vi "Actor Core.vi"(8 "error in (no error)":errorcluster, 11 "Websocket Server in":refnum<class "Websocket Server.lvclass">) -> (0 "error out":errorcluster, 3 "Websocket Server out":refnum<class "Websocket Server.lvclass">)   [LabVIEW 2016, in "Stream Mediator.lvlib" / "Websocket Server.lvclass"]
doc: "--\nCopyright © 2017 Composed SystemsI All rights reserved.\n\nAuthor: Jon McBee <jon.mcbee@composed.io>\n\nThis library is provided \"AS IS\" ,WITHOUT WARRANTIES OR\nCONDITIONS OF ANY KIND, either express or implied.\n\nComposed Systems -- composed.io\n\nStream 0.0.1.1\nJon McBee - Composed Systems\nCopyright (c) 2017, Composed Systems"
uses:
  <userlib>/Composed Systems/Stream/Mediator/Classes/Websocket Server Actor/Websocket Server/Websocket Server.lvclass
  C:/Program Files (x86)/National Instruments/LabVIEW 2016/user.lib/Composed Systems/Stream/Mediator/Classes/Mediated Asynchronous Actor/Mediated Asynchronous Actor.lvclass
  <userlib>/Composed Systems/Stream/Mediator/Classes/Message Transport Queue/Message Transport Queue.lvclass
  <userlib>/Composed Systems/Stream/Mediator/Classes/Websocket Server Actor/Websocket Server/Websocket Server.lvclass/Websocket Server.ctl
  <userlib>/Composed Systems/Stream/Mediator/Classes/Mediated Asynchronous Actor/Mediated Asynchronous Actor.lvclass
  <userlib>/Composed Systems/Stream/Mediator/Classes/Websocket Server Actor/Websocket Server Msgs/Launch Client Handler Actor Msg/Launch Client Handler Actor Msg.lvclass
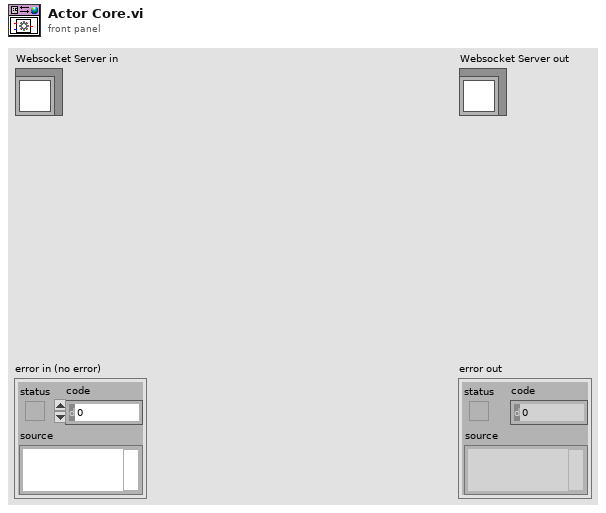
[diagram p1: front panel]
types:
  T1 = cluster{"Self Enqueuer":refnum<class "Message Transport Queue.lvclass">, "Listen Port":u16, "Listener ID":refnum<k5>}
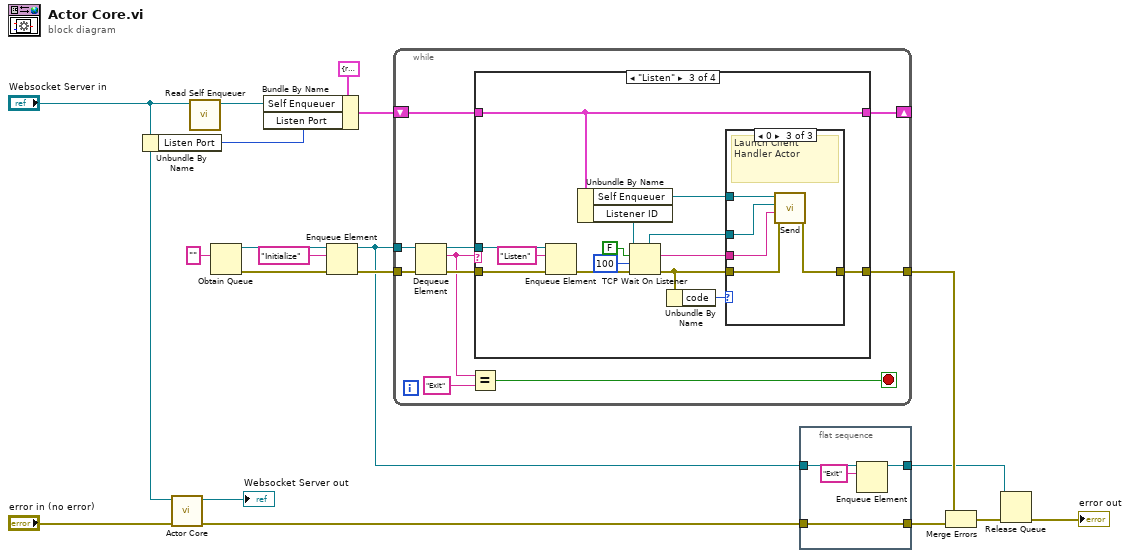
[diagram p0: block diagram]
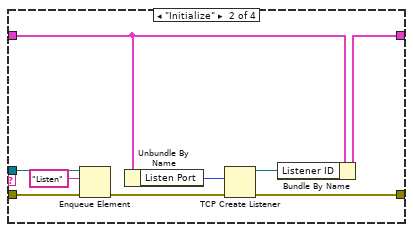
[diagram p3: hidden frame]
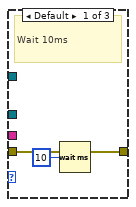
[diagram p4: hidden frame]
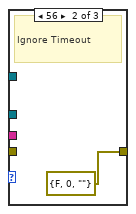
[diagram p5: hidden frame]
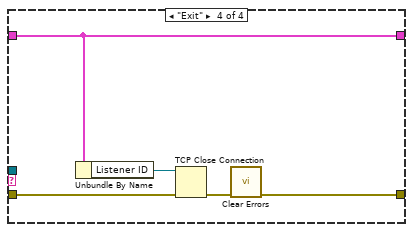
[diagram p6: hidden frame]
diagram:
  n1 = Unbundle By Name("Websocket Server in") -> ("Listen Port"=w9:u16)
  n2 = call-parent "Actor Core.vi"("error in (no error)"="error in (no error)", "Mediated Asynchronous Actor in"="Websocket Server in") -> ("error out"=w13:errorcluster, "Mediated Asynchronous Actor out"=→"Websocket Server out":refnum<class "Websocket Server.lvclass">)  [unwired: 8 in]
  n3 = call <userlib>:"Read Self Enqueuer.vi"("Mediated Asynchronous Actor in"="Websocket Server in") -> ("Self Enqueuer"=w2:refnum<class "Message Transport Queue.lvclass">)  [unwired: 10 in]
  n4 = Obtain Queue(element data type="") -> (queue out=w14:refnum<queue>, error out=w17:errorcluster)  [unwired: 4 in, 1 out]
  n5 = Bundle By Name(cluster=T1 {"Self Enqueuer"=refnum, "Listen Port"=0, "Listener ID"=refnum}, "Self Enqueuer"=w2, "Listen Port"=w9) -> (w8:T1)
  n6 = Enqueue Element(queue=w14, element="Initialize", error in (no error)=w17) -> (queue out=w11:refnum<queue>, error out=w16:errorcluster)  [unwired: 1 in, 1 out]
  n7 = while {
    tunnel: w11 -> [w29]
    tunnel: w16 -> [w28]
    shift-right: [w24] -> _
    shift-left: w8 -> [w25]
    tunnel: [w20] -> w7
    stop <- w21 stop-if-true
    n8 = Dequeue Element(queue=w29, error in (no error)=w28) -> (queue out=w27:refnum<queue>, element=w23:string, error out=w26:errorcluster)  [unwired: 1 in, 1 out]
    n9 = Equal?(x=w23, y="Exit") -> (x = y?=w21:bool)
    n10 = case shown="\"Listen\"" w23 {
      tunnel: w27 -> [_ w40 w51 _]
      tunnel: w26 -> [w30 w39 w52 w66]
      tunnel: w25 -> [w31 w33 w48 w64]
      tunnel: [w31 w32 w48 w64] -> w24
      tunnel: [w30 w36 w44 w65] -> w20
      frame "", Default {
      }
      frame "Initialize" {
        n11 = Enqueue Element(queue=w40, element="Listen", error in (no error)=w39) -> (error out=w37:errorcluster)  [unwired: 1 in, 2 out]
        n12 = Unbundle By Name(w33) -> ("Listen Port"=w35:u16)
        n13 = TCP Create Listener(8:w37, 10:w35) -> (0:w36:errorcluster, 3:w34:refnum<k5>)  [unwired: 3 in, 1 out]
        n14 = Bundle By Name(cluster=w33, "Listener ID"=w34) -> (w32:T1)
      }
      frame "Listen" {
        n15 = Enqueue Element(queue=w51, element="Listen", error in (no error)=w52) -> (error out=w49:errorcluster)  [unwired: 1 in, 2 out]
        n16 = Unbundle By Name(w48) -> ("Self Enqueuer"=w43:refnum<class "Message Transport Queue.lvclass">, "Listener ID"=w47:refnum<k5>)
        n17 = TCP Wait On Listener(8:w49, 9:100 ("timeout ms (wait forever: -1)"), 10:FALSE ("resolve remote address (T)"), 11:w47) -> (0:w45:errorcluster, 2:w42:string, 4:w41:refnum<k5>)  [unwired: 2 out]
        n18 = Unbundle By Name(w45) -> ("code"=w46:i32)
        n19 = case shown="0" w46 {
          tunnel: w45 -> [w56 _ w61]
          tunnel: [w56 errorcluster {"status"=FALSE, "code"=0, "source"=""} ("error constant") w60] -> w44
          tunnel: w43 -> [_ _ w62]
          tunnel: w42 -> [_ _ w59]
          tunnel: w41 -> [_ _ w58]
          frame Default {
            # "Wait 10ms"
            n20 = Wait (ms)(milliseconds to wait=u32 10) -> ()  [unwired: 1 out]
          }
          frame 56 {
            # "Ignore Timeout"
          }
          frame 0 {
            # "Launch Client Handler Actor"
            n21 = call <userlib>:"Send.vi"("error in (no error)"=w61, "Remote Address"=w59, "WebSocket Connection in"=w58, "Message Transport Queue"=w62) -> ("error out"=w60:errorcluster)  [unwired: 7 in]
          }
        }
      }
      frame "Exit" {
        n22 = Unbundle By Name(w64) -> ("Listener ID"=w63:refnum<k5>)
        n23 = TCP Close Connection(connection ID=w63, error in (no error)=w66) -> (error out=w67:errorcluster)  [unwired: 1 in, 1 out]
        n24 = call <vilib>:"Clear Errors.vi"("error in (no error)"=w67) -> ("error out"=w65:errorcluster)  [unwired: 5 in, 1 out]
      }
    }
  }
  n25 = flat-sequence {
    tunnel: w13 -> [w71]
    tunnel: [w71] -> w12
    tunnel: w11 -> [w70]
    tunnel: [w68] -> w4
    frame #0 {
      n26 = Enqueue Element(queue=w70, element="Exit") -> (queue out=w68:refnum<queue>)  [unwired: 2 in, 2 out]
    }
  }
  n27 = Merge Errors(w7, w12) -> (w6:errorcluster)
  n28 = Release Queue(queue=w4, error in (no error)=w6) -> (error out=→"error out":errorcluster)  [unwired: 1 in, 2 out]
